vi "construct.vi"(8 "error in (no error)":errorcluster, 9 "configuration name":string, 10 "load config file?":bool=TRUE, 11 "StimulatorDL090727DAQmx in":refnum<class "StimulatorDL090727Writer.lvclass">) -> (0 "error out":errorcluster, 3 "StimulatorDL090727DAQmx out":refnum<class "StimulatorDL090727Writer.lvclass">)   [LabVIEW 2010, in "StimulatorDL090727Writer.lvclass"]
uses:
  StimulatorDL090727Writer.lvclass
  StimulatorDL090724Scaffold/StimulatorDL090724Scaffold/Stimulator090724Scaffold.lvclass
  SignalWriter/GenericSignalWriter/GenericSignalWriter/GenericSignalWriter.lvclass
  StimulatorDL090727Writer.lvclass/StimulatorDL090727Writer.ctl
  common/classes/GenericComponent/GenericComponent/GenericComponent.lvclass
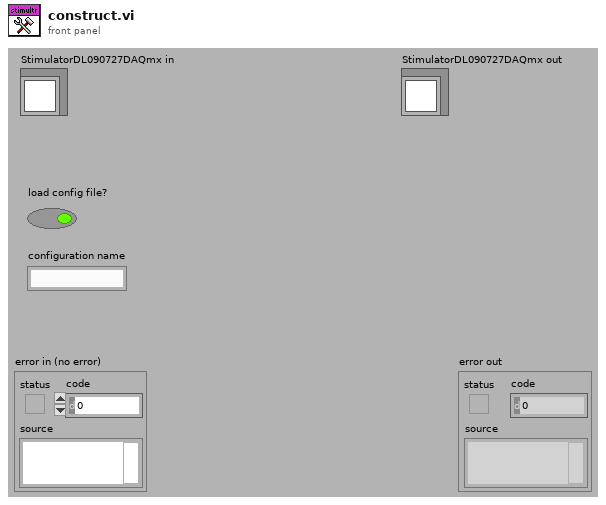
[diagram p1: front panel]
types:
  T1 = typedef "plugin_specification.ctl" = cluster{"class path":string, "configuration":string, "label":string, "settings name":string}
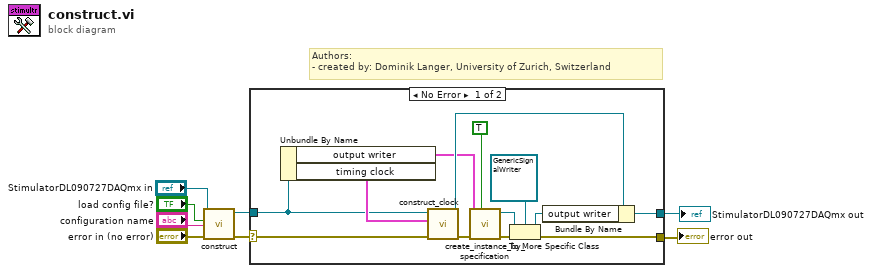
[diagram p0: block diagram]
diagram:
  # "Authors: \n- created by: Dominik Langer, University of Zurich, Switzerland"
  n1 = call-parent "construct.vi"("error in (no error)"="error in (no error)", "configuration name"="configuration name", "load config file?"="load config file?", "GenericPlugin in"="StimulatorDL090727DAQmx in") -> ("error out"=w8:errorcluster, "GenericPlugin out"=w7:refnum<class "StimulatorDL090727Writer.lvclass">)  [unwired: 6 out]
  n2 = case shown="No Error" w8 {
    selector: w8 -> [w19 w23]
    tunnel: w7 -> [w12 w22]
    tunnel: [w10 w23] -> w3
    tunnel: [w9 w22] -> w1
    frame No Error {
      n3 = Unbundle By Name(w12) -> ("output writer"=w13:T1, "timing clock"=w20:T1)
      n4 = call-dynamic "construct_clock.vi"("error in (no error)"=w19, "clock specification"=w20, "Stimulator090724Scaffold in"=w12) -> ("error out"=w17:errorcluster, "Stimulator090724Scaffold out"=w18:refnum<class "StimulatorDL090727Writer.lvclass">)  [unwired: 7 in]
      n5 = call "create_instance_by_specification.vi"("call constructor?"=TRUE, "error in (no error)"=w17, "component specification"=w13) -> ("error out"=w16:errorcluster, "GenericPlugin out"=w14:refnum<class "GenericComponent.lvclass">)  [unwired: 6 in, 1 out]
      n6 = To More Specific Class(target class=refnum<class "GenericSignalWriter.lvclass"> refnum ("GenericSignalWriter.lvclass"), reference=w14, error in=w16) -> (specific class reference=w15:refnum<class "GenericSignalWriter.lvclass">, error out=w10:errorcluster)
      n7 = Bundle By Name(cluster=w18, "output writer"=w15) -> (w9:refnum<class "StimulatorDL090727Writer.lvclass">)
    }
    frame Error {
    }
  }
  "error out" <- w3
  "StimulatorDL090727DAQmx out" <- w1
